vi "RT_Clear DMA Data.vi"(8 "error in":errorcluster, 11 "Main Data In":T1) -> (0 "error out":errorcluster, 3 "Main Data Out":T1)   [LabVIEW 2018]
uses:
  Data Def/RT_Main Data.ctl
  Data Def/RT_FPGA VI Reference.ctl
  <vilib>/Utility/error.llb/Error Cluster From Error Code.vi
  <vilib>/rvi/errors/niLvFpgaAdjustHostInterfaceError.vi
  <vilib>/rvi/interface/common/niFpgaWaitOnOcc.vi
  <vilib>/rvi/interface/nirviMethod/nirviMethod.xnode
  <vilib>/FPGAPlugInAG/Dynamic/niLvFpga_ReadFifo_Dynamic.vi
  <vilib>/rvi/errors/niLvFpgaMergeErrorWithErrorCode.vi
  <vilib>/FPGAPlugInAG/Dynamic/niLvFpga_ConfigureFifo_Dynamic.vi
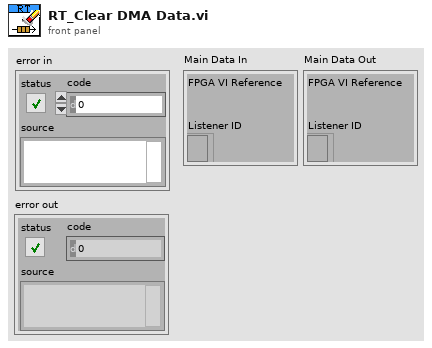
[diagram p1: front panel]
types:
  T1 = typedef "RT_Main Data.ctl" = cluster{"FPGA VI Reference":T2, "Listener ID":refnum<k5>}
  T2 = typedef "RT_FPGA VI Reference.ctl" = refnum<k20>
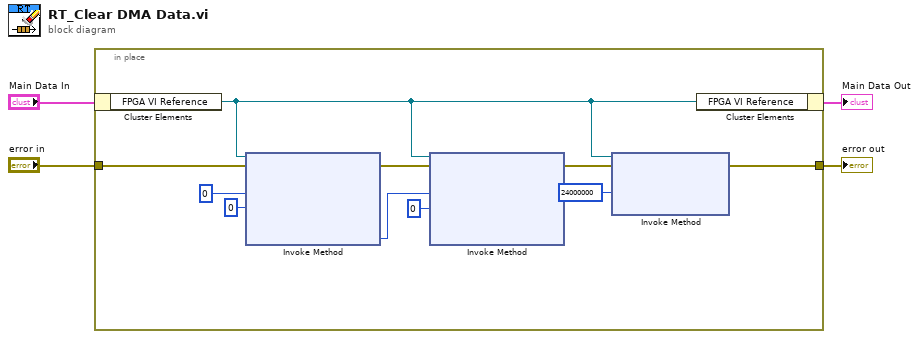
[diagram p0: block diagram]
diagram:
  n1 = in-place {
    in-place-border: "error in" -> [w7]
    in-place-border: [w5] -> w1
    n2 = in-place-cluster #1("Main Data In") -> ("FPGA VI Reference"=w6:T2)
    n3 = xnode "Invoke Method"("FPGA VI Reference In"=w6, "error in"=w7, "Number of Elements"=u32 0, "Timeout (ms)"=0) -> ("error out"=w12:errorcluster, "Elements Remaining"=w11:u32)  [unwired: 2 out]
    n4 = xnode "Invoke Method"("FPGA VI Reference In"=w6, "error in"=w12, "Number of Elements"=w11, "Timeout (ms)"=0) -> ("error out"=w10:errorcluster)  [unwired: 3 out]
    n5 = xnode "Invoke Method"("FPGA VI Reference In"=w6, "error in"=w10, "Requested Depth"=u32 24000000) -> ("error out"=w5:errorcluster)  [unwired: 2 out]
    n6 = in-place-cluster #1("FPGA VI Reference"=w6) -> (→"Main Data Out":T1)
  }
  "error out" <- w1
